vi "Begin.vi"() -> (0 "error out":errorcluster)   [LabVIEW 2018]
doc: "Called before other user functions, this VI is expected to open initial I/O refnums, load in file data, and do all program initialization. Notice that the <B>error out</B> terminal is simply used for data flow. Wiring it to other structures or subVIs ensures that this VI runs first."
uses:
  <vilib>/Rock Robotics/WPI/DriverStation/WPI_DriverStationRobotMode2.ctl
  <vilib>/Rock Robotics/WPI/Joystick/WPI_JoystickDeviceEnum.ctl
  <vilib>/Rock Robotics/SystemInterfaces/DIO/FPGA_DIOChannel.ctl
  <vilib>/Rock Robotics/SystemInterfaces/DIO/FPGA_DIOPWMChannel.ctl
  <vilib>/Rock Robotics/SystemInterfaces/AI/FPGA_AIChannel.ctl
  <vilib>/Rock Robotics/SystemInterfaces/i2clib/i2c_bus.ctl
  Drivetype.ctl
  Robot Global Data.vi
  <vilib>/Rock Robotics/Network Tables/NT Write String Array.vi
  <vilib>/Rock Robotics/WPI/Counter/WPI_CounterDigitalInputToDigitalSource.vi
  <vilib>/Rock Robotics/WPI/MotorControl/WPI_MotorControlOpen VictorSP.vi
  <vilib>/Rock Robotics/WPI/MotorControl/WPI_MotorControlOpen TalonSRX.vi
panel:
  out "Data Out":u8[](array[numeric])
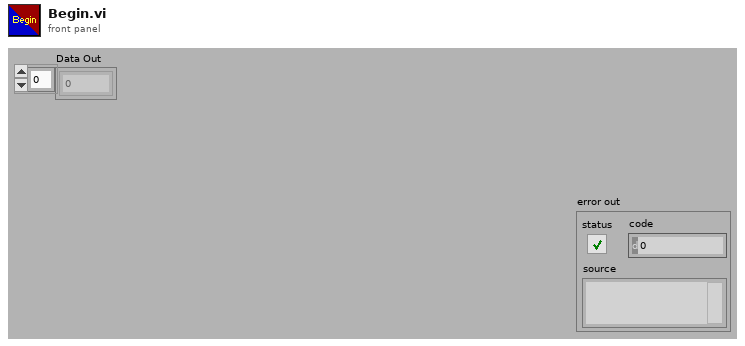
[diagram p1: front panel]
types:
  T1 = typedef "Drivetype.ctl" = enum16{"4 vitesse", "1 vitesse"}
  T2 = typedef "i2c_bus.ctl" = enum16{"I2C On-Board", "I2C MXP", "Invalid"}
  T3 = typedef "FPGA_DIOPWMChannel.ctl" = enum8{"PWM 0", "PWM 1", "PWM 2", "PWM 3", "PWM 4", "PWM 5", "PWM 6", "PWM 7", "PWM 8", "PWM 9", "PWM MXP 0", "PWM MXP 1", "PWM MXP 2", "PWM MXP 3", "PWM MXP 4", "PWM MXP 5", "PWM MXP 6", "PWM MXP 7", "PWM MXP 8", "PWM MXP 9", "Invalid"}
  T4 = typedef "FPGA_AIChannel.ctl" = enum8{"AI 0", "AI 1", "AI 2", "AI 3", "AI MXP 0", "AI MXP 1", "AI MXP 2", "AI MXP 3", "Invalid"}
  T5 = typedef "WPI_JoystickDeviceEnum.ctl" = enum16{"USB 0", "USB 1", "USB 2", "USB 3", "USB 4", "USB 5"}
  T6 = typedef "FPGA_DIOChannel.ctl" = enum8{"DIO 0", "DIO 1", "DIO 2", "DIO 3", "DIO 4", "DIO 5", "DIO 6", "DIO 7", "DIO 8", "DIO 9", "DIO MXP 0", "DIO MXP 1", "DIO MXP 2", "DIO MXP 3", "DIO MXP 4", "DIO MXP 5", "DIO MXP 6", "DIO MXP 7", "DIO MXP 8", "DIO MXP 9", "DIO MXP 10", "DIO MXP 11", "DIO MXP 12", "DIO MXP 13", "DIO MXP 14", "DIO MXP 15", "SPI Port CS1", "SPI Port CS2", "SPI Port CS3", "SPI Port MISO", "SPI Port MOSI", "Invalid"}
  T7 = typedef "WPI_DriverStationRobotMode2.ctl" = enum16{"Autonomous Disabled", "Autonomous Enabled", "Teleop Disabled", "Teleop Enabled", "Disconnected", "Finish", "Test Disabled", "Test Enabled", "Emergency Stopped"}
  T8 = typedef "WPI_MotorControlDeviceRef.ctl" = cluster{"DeviceStatus":errorcluster, "Type":T9, "PWM":cluster{"PWM Channel":T3, "DeadBand":T10}, "CAN":cluster{"Device Number":u8, "SetOutput VI Ref":variant, "GetOutput VI Ref":variant, "Enable VI Ref":variant, "Disable VI Ref":variant, "Data":variant}, "Invert":bool, "DIO PWM":cluster{"PWM \"Enable\" Channel":T3, "DIOChannel":T6, "PWM Rate":dbl}}
  T9 = typedef "WPI_MotorControlType.ctl" = enum16{"PWM", "CAN", "DIO PWM"}
  T10 = typedef "WPI_PWMDeadband.ctl" = cluster{"Name":string, "maxPositivePwm":i32, "minPositivePwm":i32, "centerPwm":i32, "maxNegativePwm":i32, "minNegativePwm":i32, "angularRange":u16}
  T11 = typedef "WPI_JoystickDevRef.ctl" = cluster{"Device":T5}
  T12 = typedef "WPI_DigitalInputDevRef.ctl" = cluster{"DevStatus":errorcluster, "DIO Channel":T6}
  T13 = typedef "FPGA_CounterEncoderSourceConvertionLVSourceType.ctl" = cluster{"DevStatus":errorcluster, "AnalogTriggerMode?":bool, "DigitalMode":cluster{"DIO Channel":T14}, "AnalogTriggerMode":cluster{"AnalogTriggerIndex":T15, "OutputType":T16}}
  T14 = typedef "FPGA_DIODigitalSourceChannel.ctl" = enum8{"DIO 0", "DIO 1", "DIO 2", "DIO 3", "DIO 4", "DIO 5", "DIO 6", "DIO 7", "DIO 8", "DIO 9", "DIO MXP 0", "DIO MXP 1", "DIO MXP 2", "DIO MXP 3", "DIO MXP 4", "DIO MXP 5", "DIO MXP 6", "DIO MXP 7", "DIO MXP 8", "DIO MXP 9", "DIO MXP 10", "DIO MXP 11", "DIO MXP 12", "DIO MXP 13", "DIO MXP 14", "DIO MXP 15", "SPI Port CS1", "SPI Port CS2", "SPI Port CS3", "SPI Port MISO", "SPI Port MOSI", "Disabled"}
  T15 = typedef "FPGA_AnalogTriggerIndex.ctl" = enum8{"Trig 0", "Trig 1", "Trig 2", "Trig 3", "Trig 4", "Trig 5", "Trig 6", "Trig 7", "Invalid"}
  T16 = typedef "FPGA_AnalogTriggerOutType.ctl" = enum16{"InWindow", "TriggerState", "Rising", "Falling"}
  T17 = typedef "WPI_EncoderDevRef.ctl" = cluster{"DevStatus":errorcluster, "EncoderIndex":T18, "CounterIndex":T19, "DistancePerCount":dbl, "Decoding Type":T20}
  T18 = typedef "FPGA_EncoderIdx.ctl" = enum8{"Enc 0", "Enc 1", "Enc 2", "Enc 3", "Enc 4", "Enc 5", "Enc 6", "Enc 7", "Invalid"}
  T19 = typedef "FPGA_CounterCtrSystemIndex.ctl" = enum8{"Ctr 0", "Ctr 1", "Ctr 2", "Ctr 3", "Ctr 4", "Ctr 5", "Ctr 6", "Ctr 7", "Invalid"}
  T20 = typedef "WPI_EncoderType.ctl" = enum16{"1x", "2x", "4x"}
  T21 = typedef "WPI_PotentiometerDevRef.ctl" = cluster{"DevStatus":errorcluster, "Analog Channel":T4, "Invert Output":bool}
  T22 = typedef "WPI_I2CDevRef.ctl" = cluster{"DevStatus":errorcluster, "Device Address":u8, "Handle":i32, "I2C Bus":T2}
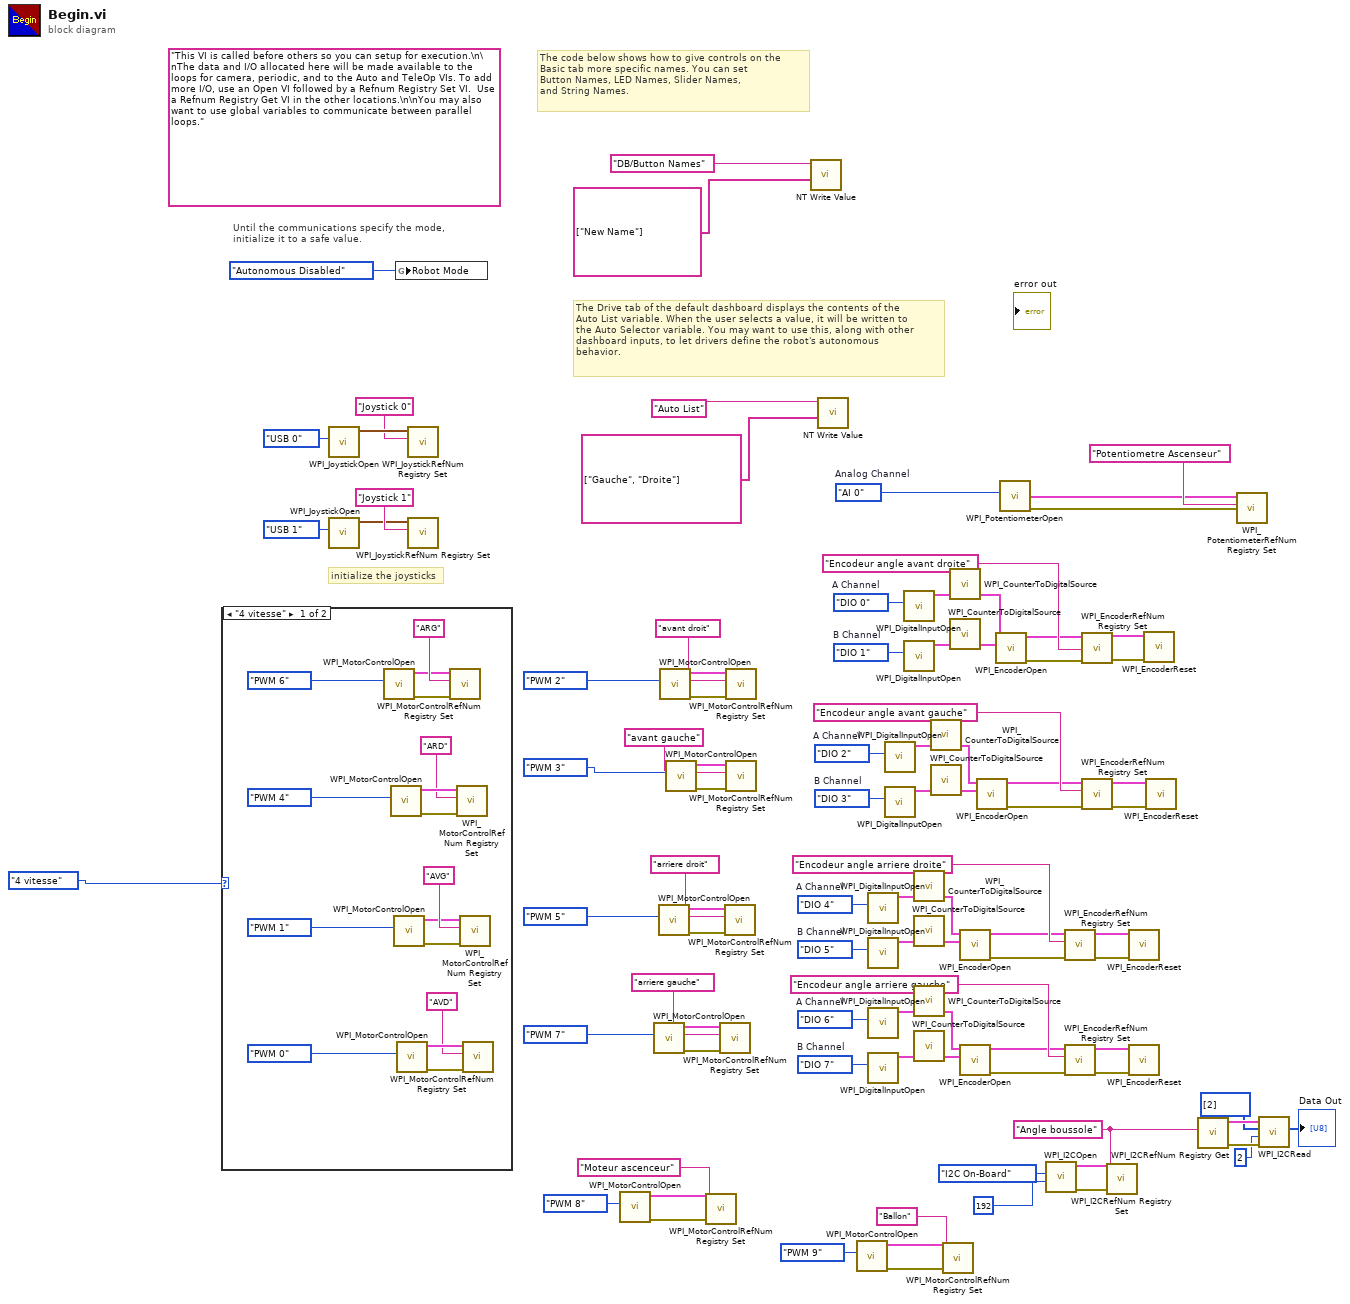
[diagram p0: block diagram]
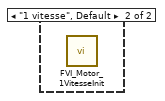
[diagram p2: hidden frame]
diagram:
  w7 = "Angle boussole" ("refnum name")
  w20 = FPGA_AIChannel."AI 0"  # Analog Channel
  w48 = FPGA_DIOChannel."DIO 7"  # B Channel
  w47 = FPGA_DIOChannel."DIO 6"  # A Channel
  w59 = FPGA_DIOChannel."DIO 5"  # B Channel
  w58 = FPGA_DIOChannel."DIO 4"  # A Channel
  w80 = FPGA_DIOChannel."DIO 3"  # B Channel
  w79 = FPGA_DIOChannel."DIO 2"  # A Channel
  w86 = FPGA_DIOChannel."DIO 1"  # B Channel
  w85 = FPGA_DIOChannel."DIO 0"  # A Channel
  (unwired) "This VI is called before others so you can setup for execution.\n\nThe data and I/O allocated here will be made available to the loops for camera, periodic, and to the Auto and TeleOp VIs. To add more I/O, use an Open VI followed by a Refnum Registry Set VI.  Use a Refnum Registry Get VI in the other locations.\n\nYou may also want to use global variables to communicate between parallel loops."
  # "The Drive tab of the default dashboard displays the contents of the\nAuto List variable. When the user selects a value, it will be written to\nthe Auto Selector variable. You may want to use this, along with other\ndashboard inputs, to let drivers define the robot's autonomous\nbehavior."
  # "The code below shows how to give controls on the\nBasic tab more specific names. You can set\nButton Names, LED Names, Slider Names,\nand String Names."
  # "initialize the joysticks"
  # "Until the communications specify the mode,\ninitialize it to a safe value."
  n1 = case shown="\"4 vitesse\"" Drivetype."4 vitesse" ("type mouvement") {
    frame "4 vitesse" {
      n2 = call-poly <vilib>:"WPI_MotorControlOpen.vi"("PWM Channel"=FPGA_DIOPWMChannel."PWM 6" ("PWM Controle roue avant")) -> ("error out"=w109:errorcluster, "MotorControlDeviceRef"=w107:T8)  [unwired: 9 in]
      n3 = call-poly <vilib>:"WPI_MotorControlOpen.vi"("PWM Channel"=FPGA_DIOPWMChannel."PWM 4" ("PWM Controle roue avant")) -> ("error out"=w104:errorcluster, "MotorControlDeviceRef"=w106:T8)  [unwired: 9 in]
      n4 = call-poly <vilib>:"WPI_MotorControlOpen.vi"("PWM Channel"=FPGA_DIOPWMChannel."PWM 1" ("PWM Controle roue avant")) -> ("error out"=w101:errorcluster, "MotorControlDeviceRef"=w99:T8)  [unwired: 9 in]
      n5 = call-poly <vilib>:"WPI_MotorControlOpen.vi"("PWM Channel"=FPGA_DIOPWMChannel."PWM 0" ("PWM Controle roue avant")) -> ("error out"=w96:errorcluster, "MotorControlDeviceRef"=w98:T8)  [unwired: 9 in]
      n6 = call <vilib>:"WPI_MotorControlRefNum Registry Set.vi"("error in (no error)"=w109, "refnum name"="ARG", "MotorControlDevRef"=w107) -> ()  [unwired: 7 in, 2 out]
      n7 = call <vilib>:"WPI_MotorControlRefNum Registry Set.vi"("error in (no error)"=w104, "refnum name"="ARD", "MotorControlDevRef"=w106) -> ()  [unwired: 7 in, 2 out]
      n8 = call <vilib>:"WPI_MotorControlRefNum Registry Set.vi"("error in (no error)"=w101, "refnum name"="AVG", "MotorControlDevRef"=w99) -> ()  [unwired: 7 in, 2 out]
      n9 = call <vilib>:"WPI_MotorControlRefNum Registry Set.vi"("error in (no error)"=w96, "refnum name"="AVD", "MotorControlDevRef"=w98) -> ()  [unwired: 7 in, 2 out]
    }
    frame "1 vitesse", Default {
      n10 = call "FVI_Motor_1VitesseInit.vi"() -> ()  [unwired: 12 in]
    }
  }
  n11 = call <vilib>:"WPI_JoystickOpen.vi"("JoystickDevice"=WPI_JoystickDeviceEnum."USB 0") -> ("JoystickDevRef"=w25:T11)  [unwired: 10 in]
  n12 = call <vilib>:"WPI_JoystickOpen.vi"("JoystickDevice"=WPI_JoystickDeviceEnum."USB 1") -> ("JoystickDevRef"=w92:T11)  [unwired: 10 in]
  n13 = global write "Robot Global Data.vi" "Robot Mode"(WPI_DriverStationRobotMode2."Autonomous Disabled" ("Robot Mode")) -> ()
  n14 = call <vilib>:"WPI_JoystickRefNum Registry Set.vi"("refnum name"="Joystick 0", "JoystickDevRef"=w25) -> ()  [unwired: 8 in, 2 out]
  n15 = call <vilib>:"WPI_JoystickRefNum Registry Set.vi"("refnum name"="Joystick 1", "JoystickDevRef"=w92) -> ()  [unwired: 8 in, 2 out]
  n16 = call-poly <vilib>:"WPI_MotorControlOpen.vi"("PWM Channel"=FPGA_DIOPWMChannel."PWM 8") -> ("error out"=w17:errorcluster, "MotorControlDeviceRef"=w18:T8)  [unwired: 9 in]
  n17 = call-poly <vilib>:"WPI_MotorControlOpen.vi"("PWM Channel"=FPGA_DIOPWMChannel."PWM 7" ("PWM Controle roue avant")) -> ("error out"=w32:errorcluster, "MotorControlDeviceRef"=w34:T8)  [unwired: 9 in]
  n18 = call-poly <vilib>:"WPI_MotorControlOpen.vi"("PWM Channel"=FPGA_DIOPWMChannel."PWM 5" ("PWM Controle roue avant")) -> ("error out"=w28:errorcluster, "MotorControlDeviceRef"=w30:T8)  [unwired: 9 in]
  n19 = call-poly <vilib>:"WPI_MotorControlOpen.vi"("PWM Channel"=FPGA_DIOPWMChannel."PWM 2" ("PWM Controle roue avant")) -> ("error out"=w67:errorcluster, "MotorControlDeviceRef"=w72:T8)  [unwired: 9 in]
  n20 = call-poly <vilib>:"WPI_MotorControlOpen.vi"("PWM Channel"=FPGA_DIOPWMChannel."PWM 3" ("PWM arrière gauche")) -> ("error out"=w70:errorcluster, "MotorControlDeviceRef"=w71:T8)  [unwired: 9 in]
  n21 = call <vilib>:"WPI_MotorControlRefNum Registry Set.vi"("error in (no error)"=w17, "refnum name"="Moteur ascenceur", "MotorControlDevRef"=w18) -> ()  [unwired: 7 in, 2 out]
  n22 = call <vilib>:"WPI_MotorControlRefNum Registry Set.vi"("error in (no error)"=w32, "refnum name"="arriere gauche", "MotorControlDevRef"=w34) -> ()  [unwired: 7 in, 2 out]
  n23 = call <vilib>:"WPI_MotorControlRefNum Registry Set.vi"("error in (no error)"=w28, "refnum name"="arriere droit", "MotorControlDevRef"=w30) -> ()  [unwired: 7 in, 2 out]
  n24 = call <vilib>:"WPI_MotorControlRefNum Registry Set.vi"("error in (no error)"=w67, "refnum name"="avant droit", "MotorControlDevRef"=w72) -> ()  [unwired: 7 in, 2 out]
  n25 = call <vilib>:"WPI_MotorControlRefNum Registry Set.vi"("error in (no error)"=w70, "refnum name"="avant gauche", "MotorControlDevRef"=w71) -> ()  [unwired: 7 in, 2 out]
  n26 = call-poly <vilib>:"NT Write Value.vi"("String Array"=string[] ["New Name"], "Name"="DB/Button Names") -> ()  [unwired: 9 in, 1 out]
  n27 = call-poly <vilib>:"NT Write Value.vi"("String Array"=string[] ["Gauche", "Droite"], "Name"="Auto List") -> ()  [unwired: 9 in, 1 out]
  n28 = call-poly <vilib>:"WPI_MotorControlOpen.vi"("PWM Channel"=FPGA_DIOPWMChannel."PWM 9") -> ("error out"=w14:errorcluster, "MotorControlDeviceRef"=w13:T8)  [unwired: 9 in]
  n29 = call <vilib>:"WPI_DigitalInputOpen.vi"("DIO Channel"=w58) -> ("DigitalInputDevRef"=w55:T12)  [unwired: 1 in, 9 out]
  n30 = call <vilib>:"WPI_DigitalInputOpen.vi"("DIO Channel"=w59) -> ("DigitalInputDevRef"=w56:T12)  [unwired: 1 in, 9 out]
  n31 = call <vilib>:"WPI_DigitalInputOpen.vi"("DIO Channel"=w47) -> ("DigitalInputDevRef"=w44:T12)  [unwired: 1 in, 9 out]
  n32 = call <vilib>:"WPI_DigitalInputOpen.vi"("DIO Channel"=w48) -> ("DigitalInputDevRef"=w45:T12)  [unwired: 1 in, 9 out]
  n33 = call <vilib>:"WPI_DigitalInputOpen.vi"("DIO Channel"=w79) -> ("DigitalInputDevRef"=w76:T12)  [unwired: 1 in, 9 out]
  n34 = call <vilib>:"WPI_DigitalInputOpen.vi"("DIO Channel"=w80) -> ("DigitalInputDevRef"=w77:T12)  [unwired: 1 in, 9 out]
  n35 = call <vilib>:"WPI_DigitalInputOpen.vi"("DIO Channel"=w85) -> ("DigitalInputDevRef"=w82:T12)  [unwired: 1 in, 9 out]
  n36 = call <vilib>:"WPI_DigitalInputOpen.vi"("DIO Channel"=w86) -> ("DigitalInputDevRef"=w83:T12)  [unwired: 1 in, 9 out]
  n37 = call-poly <vilib>:"WPI_CounterToDigitalSource.vi"("DigitalInputDevRef"=w55) -> ("Digital Source"=w54:T13)  [unwired: 6 out]
  n38 = call-poly <vilib>:"WPI_CounterToDigitalSource.vi"("DigitalInputDevRef"=w56) -> ("Digital Source"=w57:T13)  [unwired: 6 out]
  n39 = call-poly <vilib>:"WPI_CounterToDigitalSource.vi"("DigitalInputDevRef"=w44) -> ("Digital Source"=w43:T13)  [unwired: 6 out]
  n40 = call-poly <vilib>:"WPI_CounterToDigitalSource.vi"("DigitalInputDevRef"=w45) -> ("Digital Source"=w46:T13)  [unwired: 6 out]
  n41 = call-poly <vilib>:"WPI_CounterToDigitalSource.vi"("DigitalInputDevRef"=w76) -> ("Digital Source"=w75:T13)  [unwired: 6 out]
  n42 = call-poly <vilib>:"WPI_CounterToDigitalSource.vi"("DigitalInputDevRef"=w77) -> ("Digital Source"=w78:T13)  [unwired: 6 out]
  n43 = call <vilib>:"WPI_MotorControlRefNum Registry Set.vi"("error in (no error)"=w14, "refnum name"="Ballon", "MotorControlDevRef"=w13) -> ()  [unwired: 7 in, 2 out]
  n44 = call-poly <vilib>:"WPI_CounterToDigitalSource.vi"("DigitalInputDevRef"=w82) -> ("Digital Source"=w81:T13)  [unwired: 6 out]
  n45 = call-poly <vilib>:"WPI_CounterToDigitalSource.vi"("DigitalInputDevRef"=w83) -> ("Digital Source"=w84:T13)  [unwired: 6 out]
  n46 = call <vilib>:"WPI_EncoderOpen.vi"("BSource"=w57, "ASource"=w54) -> ("error out"=w51:errorcluster, "EncoderDevRef"=w52:T17)  [unwired: 6 in, 2 out]
  n47 = call <vilib>:"WPI_EncoderOpen.vi"("BSource"=w46, "ASource"=w43) -> ("error out"=w40:errorcluster, "EncoderDevRef"=w41:T17)  [unwired: 6 in, 2 out]
  n48 = call <vilib>:"WPI_EncoderOpen.vi"("BSource"=w78, "ASource"=w75) -> ("error out"=w62:errorcluster, "EncoderDevRef"=w63:T17)  [unwired: 6 in, 2 out]
  n49 = call <vilib>:"WPI_EncoderOpen.vi"("BSource"=w84, "ASource"=w81) -> ("error out"=w37:errorcluster, "EncoderDevRef"=w64:T17)  [unwired: 6 in, 2 out]
  n50 = call <vilib>:"WPI_PotentiometerOpen.vi"("Analog Channel"=w20) -> ("error out"=w21:errorcluster, "PotDevRef"=w22:T21)  [unwired: 9 in]
  n51 = call <vilib>:"WPI_I2COpen.vi"("Device Address"=u8 192, "I2C Bus"=i2c_bus."I2C On-Board") -> ("error out"=w9:errorcluster, "I2CDevRef"=w8:T22)  [unwired: 8 in]
  n52 = call <vilib>:"WPI_EncoderRefNum Registry Set.vi"("error in (no error)"=w51, "refnum name"="Encodeur angle arriere droite", "EncoderDevRef"=w52) -> ("error out"=w49:errorcluster, "EncoderDevRef"=w50:T17)  [unwired: 7 in]
  n53 = call <vilib>:"WPI_EncoderRefNum Registry Set.vi"("error in (no error)"=w40, "refnum name"="Encodeur angle arriere gauche", "EncoderDevRef"=w41) -> ("error out"=w38:errorcluster, "EncoderDevRef"=w39:T17)  [unwired: 7 in]
  n54 = call <vilib>:"WPI_EncoderRefNum Registry Set.vi"("error in (no error)"=w37, "refnum name"="Encodeur angle avant droite", "EncoderDevRef"=w64) -> ("error out"=w35:errorcluster, "EncoderDevRef"=w36:T17)  [unwired: 7 in]
  n55 = call <vilib>:"WPI_EncoderRefNum Registry Set.vi"("error in (no error)"=w62, "refnum name"="Encodeur angle avant gauche", "EncoderDevRef"=w63) -> ("error out"=w60:errorcluster, "EncoderDevRef"=w61:T17)  [unwired: 7 in]
  n56 = call <vilib>:"WPI_I2CRefNum Registry Set.vi"("error in (no error)"=w9, "refnum name"=w7, "I2CDevRef"=w8) -> ()  [unwired: 7 in, 2 out]
  n57 = call <vilib>:"WPI_EncoderReset.vi"("error in (no error)"=w49, "EncoderDevRef"=w50) -> ()  [unwired: 8 in, 2 out]
  n58 = call <vilib>:"WPI_EncoderReset.vi"("error in (no error)"=w38, "EncoderDevRef"=w39) -> ()  [unwired: 8 in, 2 out]
  n59 = call <vilib>:"WPI_EncoderReset.vi"("error in (no error)"=w35, "EncoderDevRef"=w36) -> ()  [unwired: 8 in, 2 out]
  n60 = call <vilib>:"WPI_EncoderReset.vi"("error in (no error)"=w60, "EncoderDevRef"=w61) -> ()  [unwired: 8 in, 2 out]
  n61 = call <vilib>:"WPI_I2CRefNum Registry Get.vi"("refnum name"=w7) -> ("error out"=w5:errorcluster, "I2CDevRef"=w6:T22)  [unwired: 9 in]
  n62 = call <vilib>:"WPI_PotentiometerRefNum Registry Set.vi"("error in (no error)"=w21, "refnum name"="Potentiometre Ascenseur", "PotDevRef"=w22) -> ()  [unwired: 7 in, 2 out]
  n63 = call <vilib>:"WPI_I2CRead.vi"("error in (no error)"=w5, "I2CBytesToRead"=u8 2, "I2CRegister"=u8[] [2], "I2CDevRef"=w6) -> ("Data Out"=→"Data Out":u8[])  [unwired: 5 in, 2 out]
